vi "PH_Sixpack.set Status Config changed.vi"(0 "VI in":refnum<vi>, 2 "Config changed?":bool, 5 "error in":errorcluster) -> (14 "VI out":refnum<vi>, 19 "error out":errorcluster)   [LabVIEW 2014, in "PH_Sixpack.lvlib"]
doc: "This VI sets the status if the config has changed."
uses:
  PH_Sixpack.lvlib
  PH_Sixpack.Status.ctl
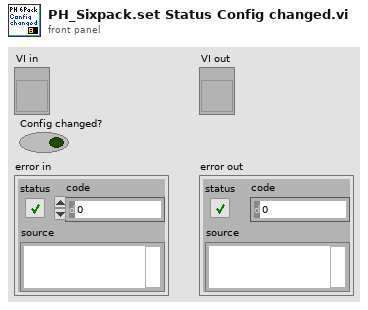
[diagram p1: front panel]
types:
  T1 = typedef "PH_Sixpack.lvlib/PH_Sixpack.Status.ctl" = enum32{"None", "Init", "Configure", "configured", "Close", "closed"}
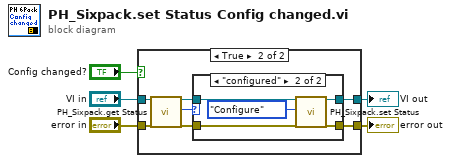
[diagram p0: block diagram]
diagram:
  n1 = case shown="True" "Config changed?" {
    tunnel: [w6 w14] -> w5
    tunnel: [w7 w13] -> w4
    tunnel: "VI in" -> [w7 w12]
    tunnel: "error in" -> [w6 w11]
    frame False {
    }
    frame True {
      n2 = call "PH_Sixpack.get Status.vi"("VI in"=w12, "error in (no error)"=w11) -> ("VI out"=w9:refnum<vi>, "Status"=w10:T1, "error out"=w8:errorcluster)  [unwired: 14 in, 1 out]
      n3 = case shown="\"configured\"" w10 {
        tunnel: w8 -> [w15 w21]
        tunnel: [w15 w20] -> w14
        tunnel: w9 -> [w16 w19]
        tunnel: [w16 w18] -> w13
        frame Default {
        }
        frame "configured" {
          n4 = call "PH_Sixpack.set Status.vi"("VI in"=w19, "Status"=PH_Sixpack.Status."Configure", "error in (no error)"=w21) -> ("VI out"=w18:refnum<vi>, "error out"=w20:errorcluster)  [unwired: 15 in]
        }
      }
    }
  }
  "error out" <- w5
  "VI out" <- w4
